vi "Get Metadata.vi"(8 "error in (no error)":errorcluster, 11 "Log Record in":refnum<class "Log Record.lvclass">) -> (0 "error out":errorcluster, 3 "Log Record out":refnum<class "Log Record.lvclass">)   [LabVIEW 2020, in "Log Record.lvclass"]
uses:
  Log Record.lvclass
  NHMFL_Core/Libraries/FAIR Data/MagX/Experiment info.ctl
  Log Record.lvclass/Log Record.ctl
panel:
  out "Data out":T1[](array[typedef])
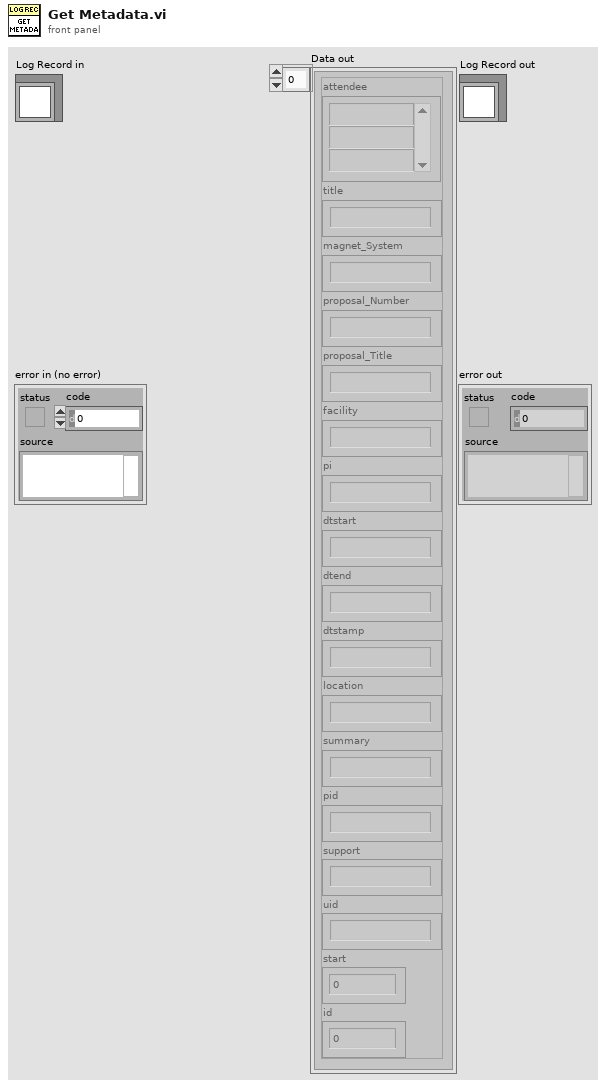
[diagram p1: front panel]
types:
  T1 = typedef "Experiment info.ctl" = cluster{"attendee":string[], "title":string, "magnet_System":string, "proposal_Number":string, "proposal_Title":string, "facility":string, "pi":string, "dtstart":string, "dtend":string, "dtstamp":string, "location":string, "summary":string, "pid":string, "support":string, "uid":string, "start":u64, "id":u64}
  T2 = typedef "Log Record Configuration.ctl" = cluster{"OSF node  ID":string, "Upload to OSF":bool, "Append to lab book ":bool, "Conection timeout":dbl, "Station":string, "Log server ":string}
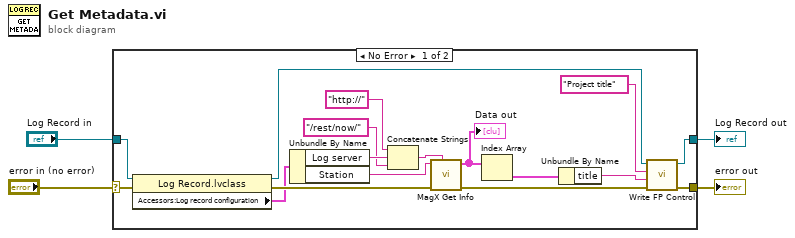
[diagram p0: block diagram]
diagram:
  n1 = case shown="No Error" "error in (no error)" {
    selector: "error in (no error)" -> [w21 w23]
    tunnel: [w17 w23] -> w3
    tunnel: [w20 w22] -> w1
    tunnel: "Log Record in" -> [w12 w22]
    frame No Error {
      n2 = property class="Log Record.lvclass"(reference=w12, error in=w21) -> (reference out=w11:refnum<class "Log Record.lvclass">, error out=w13:errorcluster, "Accessors:Log record configuration"=w10:T2)
      n3 = Unbundle By Name(w10) -> ("Log server"=w7:string, "Station"=w9:string)
      n4 = Concatenate Strings("http://" ("string"), w7, "/rest/now/" ("string")) -> (w5:string)
      n5 = call "MagX Get Info.vi"("url"=w5, "error in"=w13, "Station"=w9) -> ("error out"=w18:errorcluster, "Data out"=w16:T1[])  [unwired: 7 in]
      "Data out" <- w16
      n6 = Index Array(array=w16) -> (element=w15:T1)  [unwired: 1 in]
      n7 = Unbundle By Name(w15) -> ("title"=w14:string)
      n8 = call-dynamic "Write FP Control.vi"("error in (no error)"=w18, "Control Value"=w14, "Control Name"="Project title", "Measure Object in"=w11) -> ("error out"=w17:errorcluster, "Measure Object out"=w20:refnum<class "Log Record.lvclass">)  [unwired: 6 in]
    }
    frame Error {
    }
  }
  "error out" <- w3
  "Log Record out" <- w1
